vi "subviescrituracafe.vi"(9 "Numeric":i32, 10 "section":string) -> ()   [LabVIEW 2019, in "UI Actor.lvlib" / "UI Actor.lvclass"]
uses:
  UI Actor.lvclass
  <vilib>/Utility/config.llb/Write Key (I32).vi
  <vilib>/Utility/config.llb/NI_LVConfig.lvlib
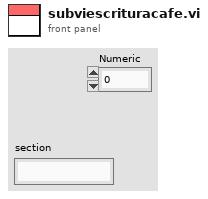
[diagram p1: front panel]
types:
  T1 = typedef "NI_LVConfig.lvlib/Config Data RefNum.ctl" = refnum<k1>
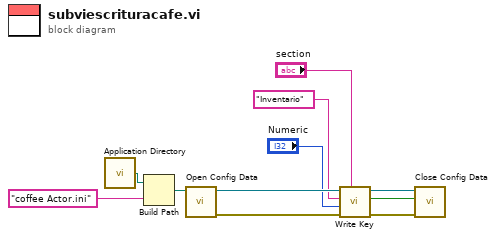
[diagram p0: block diagram]
diagram:
  n1 = call <vilib>:"Application Directory.vi"() -> ("Application Directory"=w11:path)
  n2 = Build Path(base path=w11, name or relative path="coffee Actor.ini") -> (appended path=w10:path)
  n3 = call <vilib>:"Open Config Data.vi"("configuration file path"=w10) -> ("error out"=w2:errorcluster, "refnum"=w9:T1)  [unwired: 8 in, 1 out]
  n4 = call-poly <vilib>:"Write Key.vi"("section"="section", "error in (no error)"=w2, "value"="Numeric", "key"="Inventario", "refnum"=w9) -> ("error out"=w5:errorcluster, "found?"=w4:bool, "refnum out"=w3:T1)  [unwired: 4 in]
  n5 = call <vilib>:"Close Config Data.vi"("error in (no error)"=w5, "write file if changed (T)"=w4, "refnum"=w3) -> ()  [unwired: 7 in, 2 out]
